vi "FindRect.vi"(0 "Image In":T1, 1 "Low pass/High pass (Low pass) (FFT Filter 2)":bool, 2 "Truncation Frequency % (FFT Filter 2)":sgl=5.0, 7 "error in":errorcluster) -> (20 "Image Out":T1, 21 "Centroid (Centroid 1)":cluster{"X Centroid":sgl, "Y Centroid":sgl} {"Y Centroid" format="%.2f"; "X Centroid" format="%.2f"}, 27 "error out":errorcluster)   [LabVIEW 2020]
uses:
  <vilib>/vision/Image Controls.llb/IMAQ Image.ctl
  <vilib>/vision/NI_Vision_Development_Module.lvlib
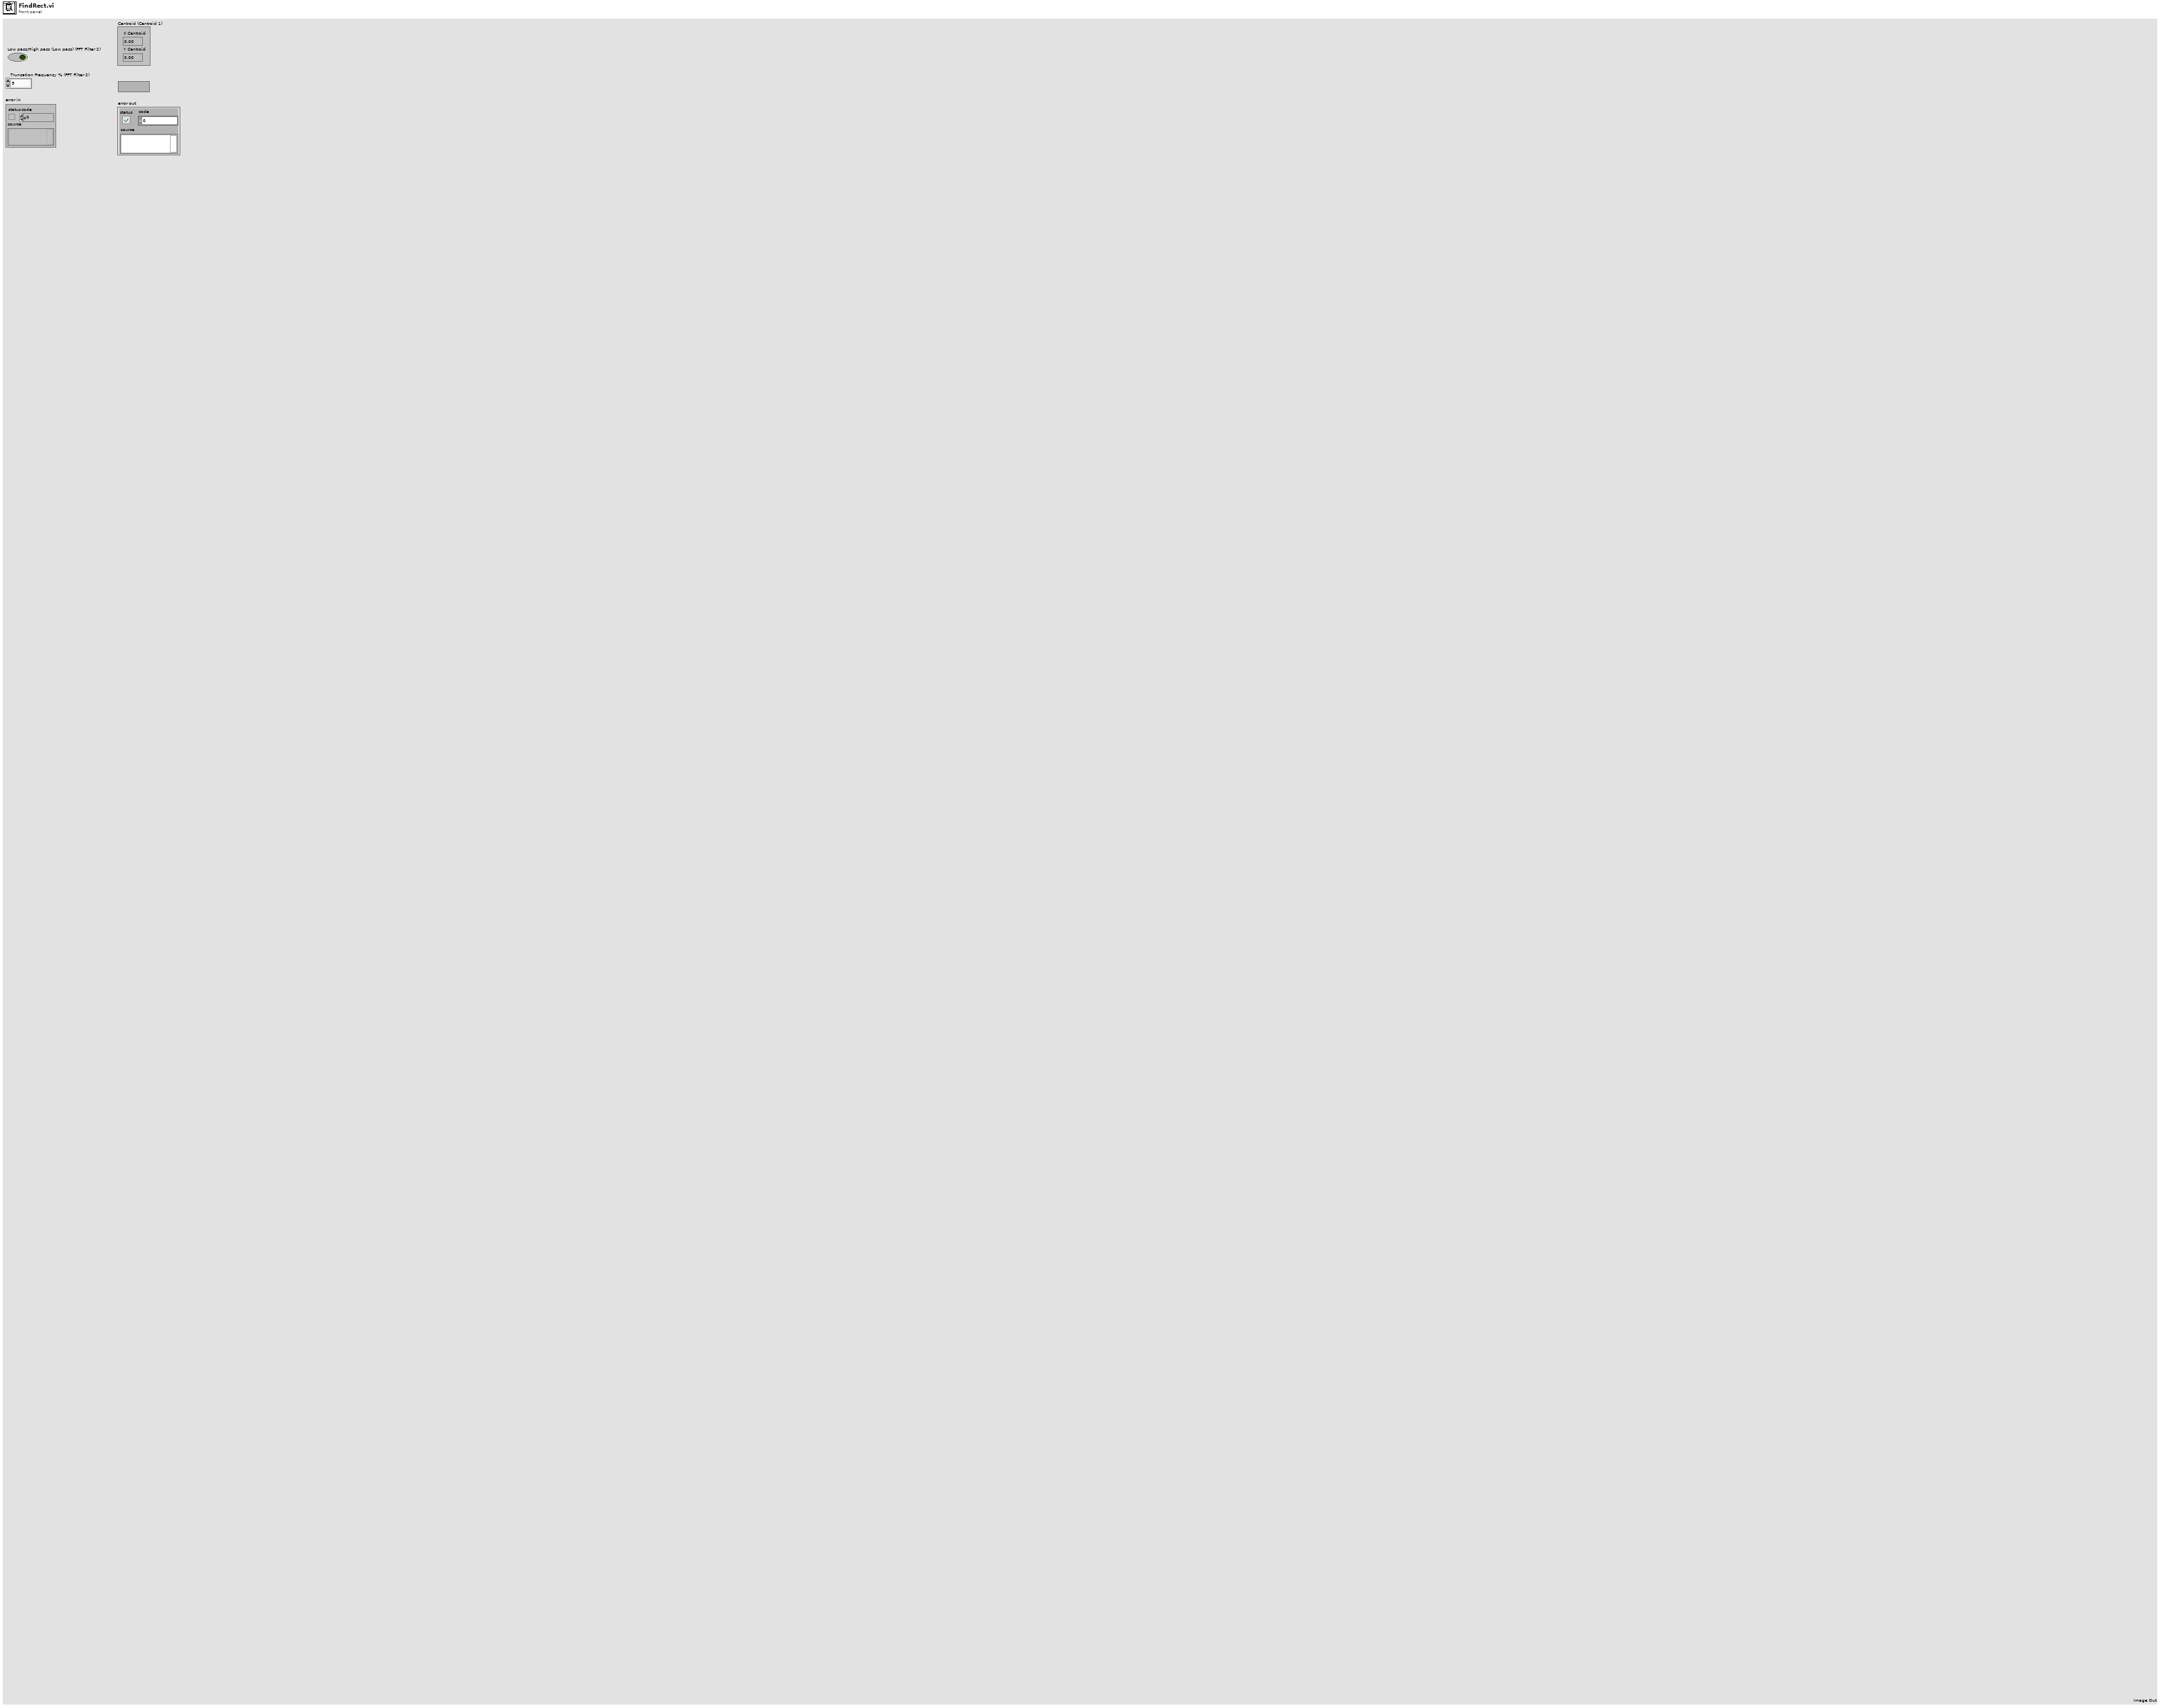
[diagram p1: front panel]
types:
  T1 = typedef "IMAQ Image.ctl" = refnum<image>
  T2 = typedef "Image Type" = u32
  T3 = cluster{"Global Rectangle":cluster{"x1Left":i32, "y1Top":i32, "x2Right":i32, "y2Bottom":i32}, "Centroid":cluster{"x":sgl, "y":sgl}, "Object Size":u32, "Score":dbl}[]
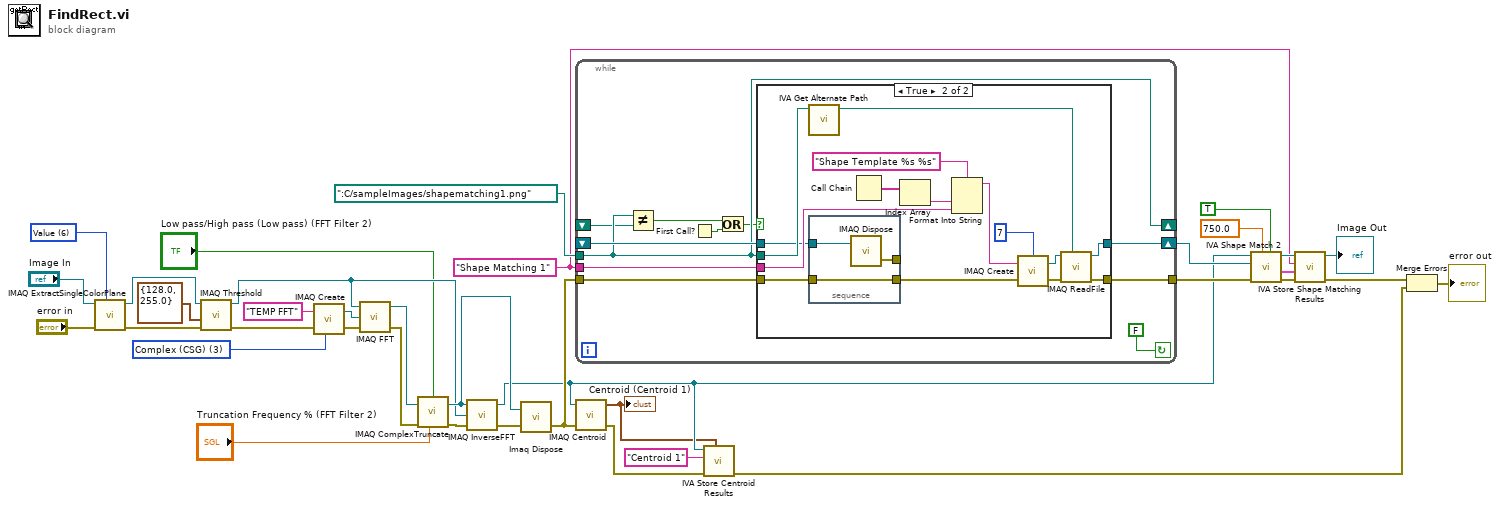
[diagram p0: block diagram]
diagram:
  w10 = "Shape Matching 1" ("Step Name")
  w19 = T2 3 items=["Grayscale (U8)", "Grayscale (I16)", "Grayscale (SGL)", "Complex (CSG)", "RGB (U32)", "HSL (U32)", "RGB (U64)", "Grayscale (U16)"] ("Image Type")
  w37 = 6 items=["Red", "Green", "Blue", "Hue", "Saturation", "Luminance", "Value", "Intensity"] ("Color Plane")
  n1 = call "IMAQ ExtractSingleColorPlane"("Color Plane"=w37, "error in (no error)"="error in", "Image Src"="Image In") -> ("error out"=w32:errorcluster, "Image Dst Out"=w33:T1)  [unwired: 1 in, 6 out]
  n2 = call "IMAQ Threshold"("error in (no error)"=w32, "Range"=cluster{"Lower value":sgl, "Upper value":sgl} {"Lower value"=128.0, "Upper value"=255.0}, "Image Src"=w33) -> ("error out"=w23:errorcluster, "Image Dst Out"=w22:T1)  [unwired: 3 in, 4 out]
  n3 = call "IMAQ Create"("Image Name"="TEMP FFT", "Image Type"=w19, "error in (no error)"=w23) -> ("New Image"=w30:T1, "error out"=w24:errorcluster)  [unwired: 1 in, 1 out]
  n4 = call "IMAQ FFT"("error in (no error)"=w24, "Image Dst"=w30, "Image Src"=w22) -> ("error out"=w28:errorcluster, "Image Dst Out"=w29:T1)  [unwired: 1 out]
  n5 = call "IMAQ ComplexTruncate"("error in (no error)"=w28, "Truncation Frequency %"="Truncation Frequency % (FFT Filter 2)", "Image Src"=w29, "Low pass/High pass (Low pass)"="Low pass/High pass (Low pass) (FFT Filter 2)") -> ("error out"=w26:errorcluster, "Image Dst Out"=w27:T1)  [unwired: 1 in, 2 out]
  n6 = call "IMAQ InverseFFT"("error in (no error)"=w26, "Image Dst"=w22, "Image Src"=w27) -> ("error out"=w25:errorcluster, "Image Dst Out"=w7:T1)  [unwired: 1 out]
  n7 = call "Imaq Dispose"("Image"=w27, "error in (no error)"=w25) -> ("error out"=w9:errorcluster)  [unwired: 1 in, 3 out]
  n8 = while {
    shift-right: [w48] -> w11
    shift-left: _ -> [w47]
    tunnel: [w45] -> w12
    tunnel: w9 -> [w44]
    tunnel: path ":C/sampleImages/shapematching1.png" ("Template Path") -> [w42]
    tunnel: w10 -> [w43]
    shift-right: [w42] -> _
    shift-left: _ -> [w41]
    stop <- FALSE continue-if-true
    n9 = Not Equal?(x=w42, y=w41) -> (x != y?=w39:bool)
    n10 = First Call?() -> (First Call?: T/F=w40:bool)
    n11 = Or(x=w39, y=w40) -> (x .or. y?=w38:bool)
    n12 = case shown="True" w38 {
      tunnel: [w50 w62] -> w48
      tunnel: w47 -> [w50 w53]
      tunnel: [w49 w60] -> w45
      tunnel: w44 -> [w49 w52]
      tunnel: w42 -> [_ w55]
      tunnel: w43 -> [_ w56]
      frame False {
      }
      frame True {
        n13 = call <vilib>:"IVA Get Alternate Path.vi"("Path In"=w55) -> ("Path Out"=w54:path)  [unwired: 10 out]
        n14 = stacked-sequence {
          tunnel: w53 -> [w68]
          tunnel: w52 -> [w67]
          tunnel: [w67] -> w51
          tunnel: [w66] -> _
          frame #0 {
            n15 = call "IMAQ Dispose"("Image"=w68) -> ("error out"=w66:errorcluster)  [unwired: 2 in, 3 out]
          }
        }
        n16 = Call Chain() -> (call chain=w58:string[])
        n17 = Index Array(array=w58) -> (element=w57:string)  [unwired: 1 in]
        n18 = Format Into String(format string="Shape Template %s %s" ("Image Name"), w57, w56) -> (resulting string=w65:string)  [unwired: 2 in, 1 out]
        n19 = call "IMAQ Create"("Border Size"=7, "Image Name"=w65, "error in (no error)"=w51) -> ("New Image"=w63:T1, "error out"=w61:errorcluster)  [unwired: 1 in, 1 out]
        n20 = call "IMAQ ReadFile"("File Path"=w54, "error in (no error)"=w61, "Image"=w63) -> ("error out"=w60:errorcluster, "Image Out"=w62:T1)  [unwired: 2 in, 5 out]
      }
    }
  }
  n21 = call "IMAQ Centroid"("error in (no error)"=w9, "Image"=w7) -> ("error out"=w8:errorcluster, "Centroid"=w5:cluster{"X Centroid":sgl, "Y Centroid":sgl})  [unwired: 1 in, 1 out]
  "Centroid (Centroid 1)" <- w5
  n22 = call <vilib>:"IVA Store Centroid Results.vi"("Centroid in"=w5, "error in (no error)"=w8, "Step Name"="Centroid 1", "Image in"=w7) -> ("error out"=w1:errorcluster)  [unwired: 7 out]
  n23 = call <vilib>:"IVA Shape Match 2.vi"("Scale Invariance"=TRUE, "Minimal Score"=750.0, "error in (no error)"=w12, "Template"=w11, "Image Src"=w7) -> ("error out"=w16:errorcluster, "Shape Report"=w15:T3, "Image Out"=w14:T1)  [unwired: 4 out]
  n24 = call <vilib>:"IVA Store Shape Matching Results.vi"("error in (no error)"=w16, "Shape Report"=w15, "Step Name"=w10, "Image in"=w14) -> ("error out"=w2:errorcluster, "Image dup"=→"Image Out":T1)  [unwired: 6 out]
  n25 = Merge Errors(w2, w1) -> (→"error out":errorcluster)
